vi "SetClockHW.vi"(8 "error in (no error)":errorcluster, 11 "BME_DG_Base in":refnum<class "BME_DG_Base.lvclass">) -> (0 "error out":errorcluster, 3 "BME_DG_Base out":refnum<class "BME_DG_Base.lvclass">)   [LabVIEW 2009, in "BME_DG_Base.lvclass"]
uses:
  BME_DG_Base.lvclass
  BME_DG_Base.lvclass/BME_DG_Base.ctl
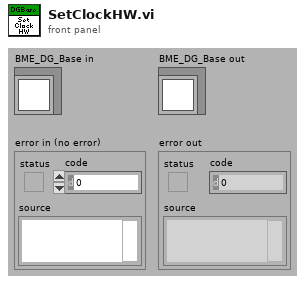
[diagram p1: front panel]
types:
  T1 = typedef "ClockSource.ctl" = i32
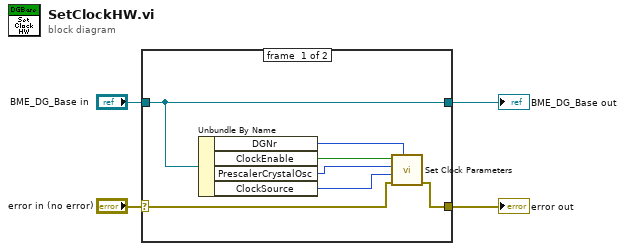
[diagram p0: block diagram]
diagram:
  n1 = case shown="No Error" "error in (no error)" {
    selector: "error in (no error)" -> [w6 w13]
    tunnel: [w5 w13] -> w3
    tunnel: [w11 w12] -> w1
    tunnel: "BME_DG_Base in" -> [w11 w12]
    frame #0 {
      n2 = Unbundle By Name(w11) -> ("DGNr"=w9:i32, "ClockEnable"=w10:bool, "PrescalerCrystalOsc"=w8:u32, "ClockSource"=w7:T1)
      n3 = call "Set Clock Parameters.vi"("DG Number"=w9, "error in (no error)"=w6, "Clock Source"=w7, "Ocillator Divide By"=w8, "Clock\nEnable"=w10) -> ("error out"=w5:errorcluster)  [unwired: 6 in]
    }
    frame #1 {
    }
  }
  "error out" <- w3
  "BME_DG_Base out" <- w1
